vi "sub_distance_processing.vi"(0 "Magnitude high":dbl[](array[numeric]), 1 "Calibration":T2 {"r bias" format="%_3p"; "Ks" format="%#_3p"}, 3 "Measurements In":T1 {"RMS" format="%#_3p"; "Relative" format="%.4f"; "Ref distance" format="%.3f"; "DC" format="%.3f"}, 5 "Magnitude low":dbl, 9 "Modulation info":T3 {"Hi channels at low" min=0 step=1; "Low carriers" format="%#_6p"; "High carriers" format="%#_6p"}, 11 "Reset":bool, 12 "Output options":T4={"Source"=enum."X", "Sensor"=enum."X", "Sense"=FALSE, "Distance"=FALSE, "LF corner"=0.0, "RMS Tc"=5.0}, 13 "Reset RMS":bool, 14 "Time Stamp":timestamp) -> (4 "Measurements out":T1 {"RMS" format="%#_3p"; "Relative" format="%.4f"; "Ref distance" format="%.3f"; "DC" format="%.3f"}, 6 "Mean level":dbl[](array[numeric]), 10 "Chart display":waveform(dbl)[](array[waveform]), 15 "Distance high":dbl[](array[numeric]))   [LabVIEW 2014]
uses:
  output_options.ctl
  coupling_selector.ctl
  modulation_info.ctl
  measurements.ctl
  calibration.ctl
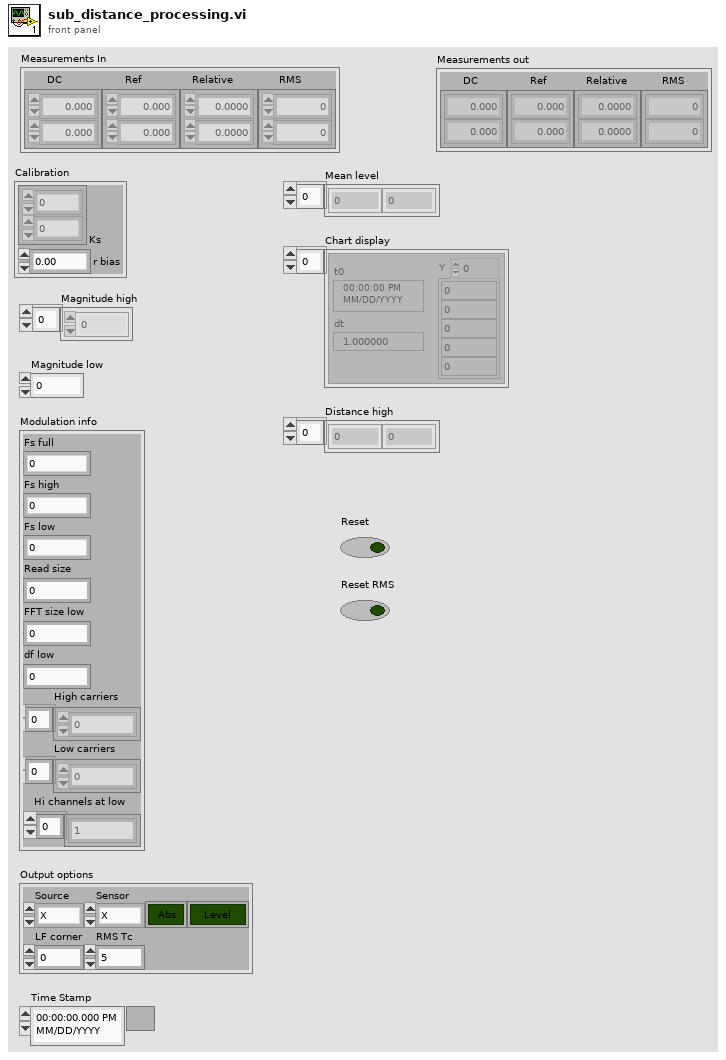
[diagram p1: front panel]
types:
  T1 = typedef "measurements.ctl" = cluster{"DC":dbl[], "Ref distance":dbl[], "Relative":dbl[], "RMS":dbl[]}
  T2 = typedef "calibration.ctl" = cluster{"Ks":dbl[], "r bias":dbl}
  T3 = typedef "modulation_info.ctl" = cluster{"Fs full":dbl, "Fs high":dbl, "Fs low":dbl, "Read size":i32, "FFT size low":i32, "df low":dbl, "High carriers":dbl[], "Low carriers":dbl[], "Hi channels at low":i32[]}
  T4 = typedef "output_options.ctl" = cluster{"Source":T5, "Sensor":T5, "Sense":bool, "Distance":bool, "LF corner":dbl, "RMS Tc":dbl}
  T5 = typedef "coupling_selector.ctl" = enum16{"X", "Y", "Z", "Vector"}
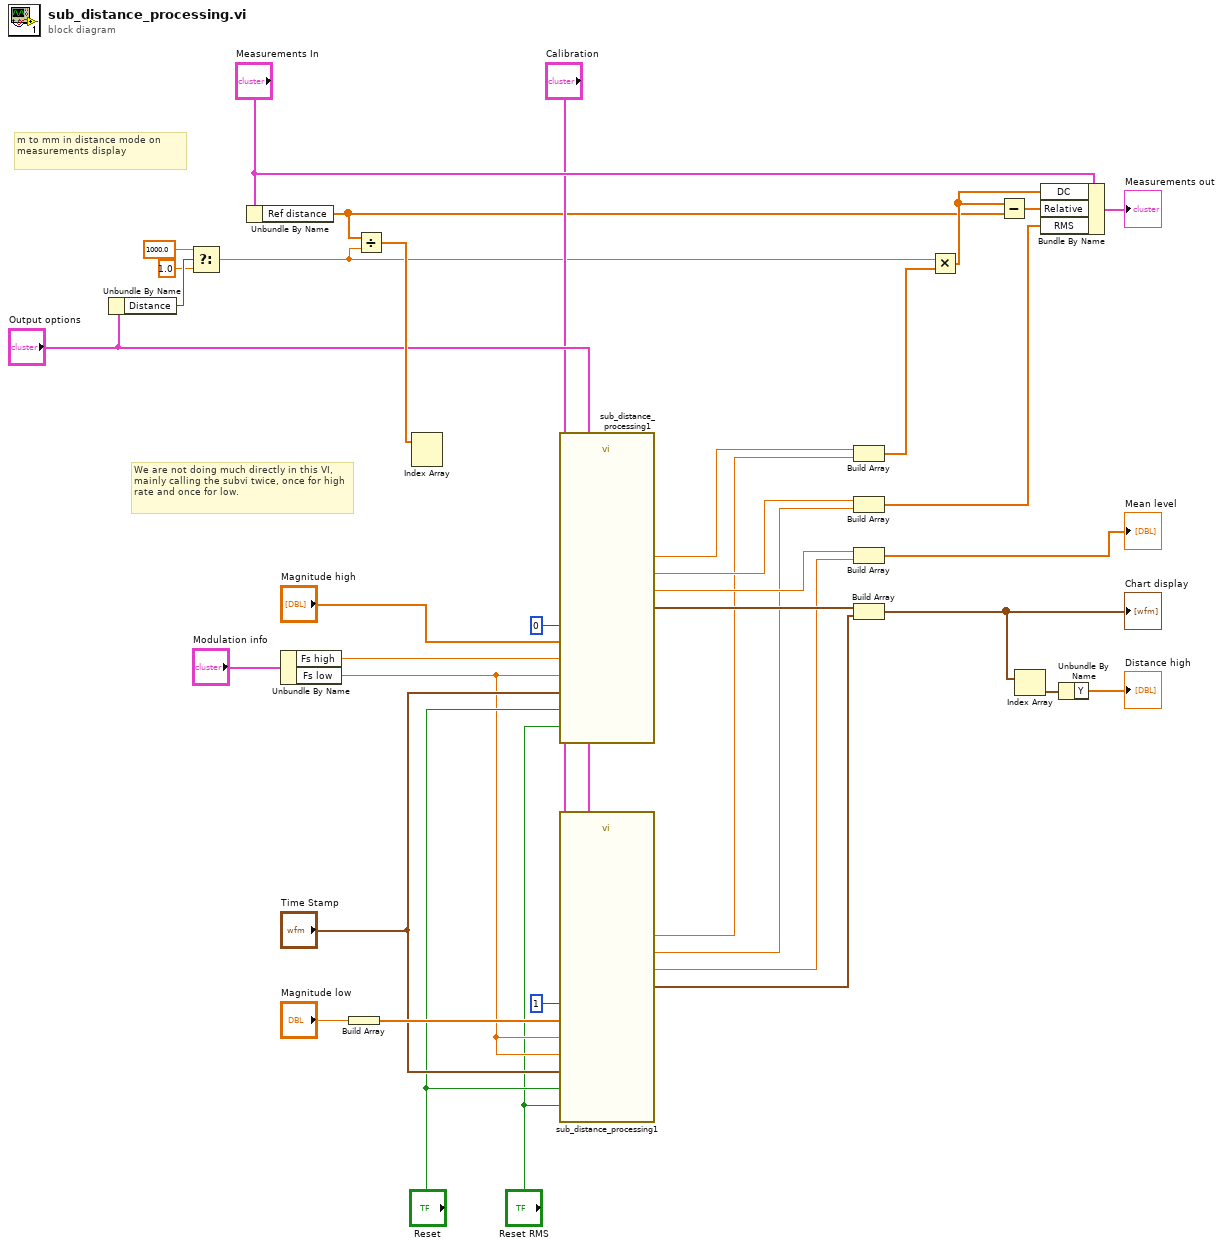
[diagram p0: block diagram]
diagram:
  # "We are not doing much directly in this VI, mainly calling the subvi twice, once for high rate and once for low."
  # "m to mm in distance mode on measurements display"
  n1 = Unbundle By Name("Output options") -> ("Distance"=w37:bool)
  n2 = Select(t=1000.0, s=w37, f=1.0) -> (s? t:f=w4:dbl)
  n3 = Unbundle By Name("Measurements In") -> ("Ref distance"=w3:dbl[])
  n4 = Unbundle By Name("Modulation info") -> ("Fs high"=w17:dbl, "Fs low"=w11:dbl)
  n5 = Build Array("Magnitude low") -> (w14:dbl[])
  n6 = Divide(x=w3, y=w4) -> (x/y=w18:dbl[])
  n7 = Index Array(array=w18) -> ()  [unwired: 2 in, 2 out]
  n8 = call "sub_distance_processing1.vi"("Calibration"="Calibration", "Reset RMS"="Reset RMS", "Output options"="Output options", "High/low index"=0, "Magnitude"="Magnitude high", "Fs low"=w11, "Fs"=w17, "Reset"="Reset", "Time Stamp"="Time Stamp") -> ("RMS"=w19:dbl, "DC"=w22:dbl, "Mean level"=w26:dbl, "Waveform"=w24:waveform(dbl))  [unwired: 3 in]
  n9 = call "sub_distance_processing1.vi"("Calibration"="Calibration", "Reset RMS"="Reset RMS", "Output options"="Output options", "High/low index"=1, "Magnitude"=w14, "Fs low"=w11, "Fs"=w11, "Reset"="Reset", "Time Stamp"="Time Stamp") -> ("RMS"=w7:dbl, "DC"=w8:dbl, "Mean level"=w6:dbl, "Waveform"=w5:waveform(dbl))  [unwired: 3 in]
  n10 = Build Array(w22, w8) -> (w21:dbl[])
  n11 = Build Array(w19, w7) -> (w2:dbl[])
  n12 = Build Array(w26, w6) -> (→"Mean level":dbl[])
  n13 = Build Array(w24, w5) -> (w23:waveform(dbl)[])
  "Chart display" <- w23
  n14 = Multiply(x=w4, y=w21) -> (x*y=w36:dbl[])
  n15 = Subtract(x=w36, y=w3) -> (x-y=w35:dbl[])
  n16 = Index Array(array=w23) -> (element=w31:waveform(dbl))  [unwired: 1 in]
  n17 = Bundle By Name(cluster="Measurements In", "DC"=w36, "Relative"=w35, "RMS"=w2) -> (→"Measurements out":T1)
  n18 = Unbundle By Name(w31) -> ("Y"=→"Distance high":dbl[])
